vi "SetText.vi"(8 "error in (no error)":errorcluster, 10 "Text":string, 11 "Heading in":refnum<class "Heading.lvclass">) -> (0 "error out":errorcluster, 3 "Heading out":refnum<class "Heading.lvclass">)   [LabVIEW 2021]
uses:
  Heading.lvclass
  C:/GitHub/Markdown/src/Markdown/Markdown.lvclass
  C:/GitHub/Markdown/src/Markdown/Heading/Heading.lvclass
  C:/GitHub/Markdown/src/Markdown/IRenderable/IRenderable.lvclass
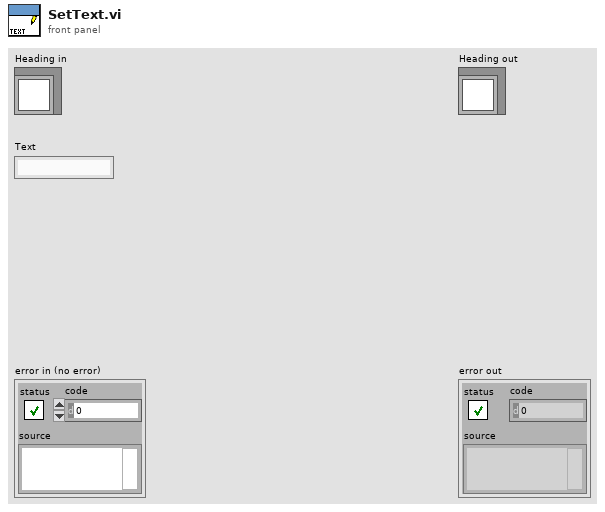
[diagram p1: front panel]
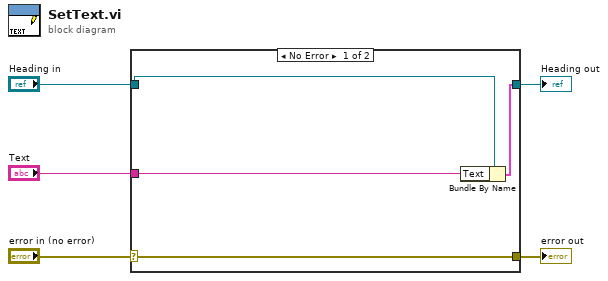
[diagram p0: block diagram]
diagram:
  n1 = case shown="No Error" "error in (no error)" {
    selector: "error in (no error)" -> [w9 w10]
    tunnel: [w9 w10] -> w4
    tunnel: [w7 w11] -> w2
    tunnel: "Heading in" -> [w8 w11]
    tunnel: "Text" -> [w6 _]
    frame No Error {
      n2 = Bundle By Name(cluster=w8, "Text"=w6) -> (w7:cluster{})
    }
    frame Error {
    }
  }
  "error out" <- w4
  "Heading out" <- w2
